vi "CVT1NamedWriteTest.vi"() -> (3 "Unit Test Framework Results":T1)   [LabVIEW 2013, in "UnitTests.lvlib"]
uses:
  UnitTests.lvlib
  <vilib>/utf/common/utf_test_result_troll.ctl
  <vilib>/utf/common/utf_test_result.ctl
  <vilib>/utf/common/utf_test_result_failure.ctl
  <vilib>/utf/common/utf_test_comparison_operators.ctl
  <vilib>/utf/common/utf_vi_tag.ctl
  <vilib>/NI/Current Value Table/Write.vi
  <vilib>/NI/Current Value Table/DataTypes/I32_Write.vi
  <vilib>/NI/Current Value Table/Read.vi
  <vilib>/NI/Current Value Table/DataTypes/I32_Read.vi
  <vilib>/NI/Current Value Table/Type to Enum.vi
  <vilib>/NI/Current Value Table/DataTypes/I32_Type To Enum.vi
  <vilib>/NI/Current Value Table/Compatibility/TagConverter.vi
  <vilib>/NI/Current Value Table/Create Tags.vi
  <vilib>/NI/Current Value Table/FGVs/CVT Globals.vi
  <vilib>/NI/Current Value Table/FGVs/Tag Memory.vi
  <vilib>/NI/Current Value Table/Memory Block.vi
  <vilib>/NI/Current Value Table/DataTypes/I32_Memory Block.vi
  <vilib>/utf/NI_UnitTestFramework.lvlib
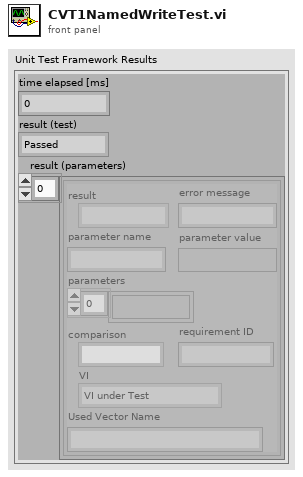
[diagram p1: front panel]
types:
  T1 = typedef "NI_UnitTestFramework.lvlib/utf_test_result_troll.ctl" = cluster{"time elapsed [ms]":u32, "result (test)":T2, "result (parameters)":T3[]}
  T2 = typedef "NI_UnitTestFramework.lvlib/utf_test_result.ctl" = enum16{"Passed", "Failed", "Error", "Skipped", "Not Processed"}
  T3 = typedef "NI_UnitTestFramework.lvlib/utf_test_result_failure.ctl" = cluster{"result":T2, "error message":string, "parameter name":string, "parameter value":variant, "parameters":variant[], "comparison":T4, "requirement ID":string, "VI":T5, "Used Vector Name":string}
  T4 = typedef "NI_UnitTestFramework.lvlib/utf_test_comparison_operators.ctl" = enum16{"=", "!=", ">", ">=", "<", "<=", "range", "symmetric tolerance", "asymmetric tolerance", "string contains", "string not contain", "array size", "string length", "array range", "by element", "array range (limit array)", "user-defined", "array contains", "array not contain", "vector length", "= (elm)", "!= (elm)", "= (case insensitive)", "!= (case insensitive)"}
  T5 = typedef "NI_UnitTestFramework.lvlib/utf_vi_tag.ctl" = enum16{"Setup VI", "VI under Test", "Teardown VI"}
  T6 = typedef "cvt_Tag Configuration.ctl" = cluster{"Name":string, "Data Type":T7, "Array":bool, "Size":u32, "Default":string, "Enum":string[], "Description":string}
  T7 = typedef "cvt_Data Types.ctl" = enum16{"Bool", "U8", "I32", "Double", "String", "Enum"}
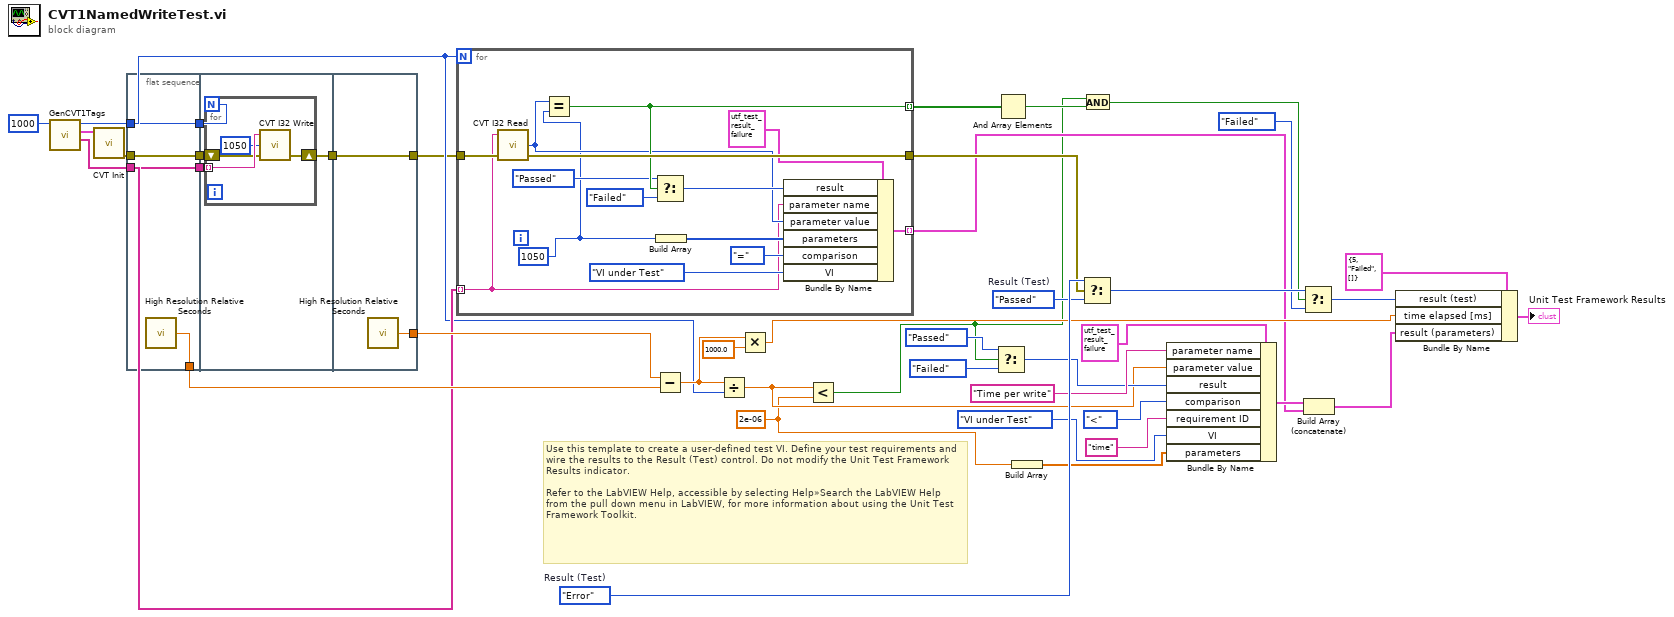
[diagram p0: block diagram]
diagram:
  w5 = 2e-06 ("y")
  w36 = utf_test_result."Error"  # Result (Test)
  w35 = utf_test_result."Passed"  # Result (Test)
  # "Use this template to create a user-defined test VI. Define your test requirements and wire the results to the Result (Test) control. Do not modify the Unit Test Framework Results indicator. \n\nRefer to the LabVIEW Help, accessible by selecting Help»Search the LabVIEW Help from the pull down menu in LabVIEW, for more information about using the Unit Test Framework Toolkit."
  n1 = call "GenCVT1Tags.vi"("Number of Tags in"=1000) -> ("Names"=w21:string[], "Tags"=w29:T6[], "Number of Tags out"=w20:i32)  [unwired: 8 in]
  n2 = call <vilib>:"CVT Init.vi"("Tag List"=w29) -> ("error out"=w28:errorcluster)  [unwired: 10 in]
  n3 = flat-sequence {
    tunnel: [w45] -> w38
    tunnel: w28 -> [w42]
    tunnel: [w44] -> w27
    tunnel: w20 -> [w44]
    tunnel: w21 -> [w43]
    tunnel: [w43] -> w26
    tunnel: [w42] -> w25
    tunnel: w27 -> [w49]
    tunnel: w26 -> [w48]
    tunnel: w25 -> [w47]
    tunnel: [w46] -> w24
    tunnel: [w55] -> w39
    tunnel: w24 -> [w54]
    tunnel: [w54] -> w19
    frame #0 {
      n4 = call <vilib>:"High Resolution Relative Seconds.vi"() -> ("relative seconds"=w45:dbl)
    }
    frame #1 {
      n5 = for {
        N: w49 -> [_]
        tunnel: w48 -> [w53] mode=indexing
        shift-right: [w51] -> w46
        shift-left: w47 -> [w52]
        n6 = call <vilib>:"CVT I32 Write.vi"("error in (no error)"=w52, "Value"=1050, "Tag Name"=w53) -> ("error out"=w51:errorcluster)  [unwired: 2 in]
      }
    }
    frame #2 {
      n7 = call <vilib>:"High Resolution Relative Seconds.vi"() -> ("relative seconds"=w55:dbl)
    }
  }
  n8 = for {
    N: w20 -> [_]
    tunnel: w21 -> [w57] mode=indexing
    tunnel: w19 -> [w69]
    tunnel: [w68] -> w18
    tunnel: [w65] -> w17 mode=indexing
    tunnel: [w61] -> w3 mode=indexing
    w56 = 1050 ("Value")
    n9 = call <vilib>:"CVT I32 Read.vi"("error in (no error)"=w69, "Tag Name"=w57) -> ("error out"=w68:errorcluster, "Value"=w58:i32)  [unwired: 2 in]
    n10 = Equal?(x=w58, y=w56) -> (x = y?=w65:bool)
    n11 = Select(t=utf_test_result."Passed" ("result"), s=w65, f=utf_test_result."Failed" ("result")) -> (s? t:f=w62:T2)
    n12 = Build Array(w56) -> (w59:i32[])
    n13 = Bundle By Name(cluster=T3 {"result"=enum."Passed", "error message"="", "parameter name"="", "parameter value"=variant, "parameters"=[], "comparison"=enum."=", "requirement ID"="", "VI"=enum."Setup VI", "Used Vector Name"=""} ("Unit Test Framework - result (parameters)"), "result"=w62, "parameter name"=w57, "parameter value"=w58, "parameters"=w59, "comparison"=utf_test_comparison_operators."=", "VI"=utf_vi_tag."VI under Test") -> (w61:T3)
  }
  n14 = Subtract(x=w39, y=w38) -> (x-y=w23:dbl)
  n15 = Divide(x=w23, y=w20) -> (x/y=w8:dbl)
  n16 = Multiply(x=w23, y=1000.0) -> (x*y=w30:dbl)
  n17 = Less?(x=w8, y=w5) -> (x < y?=w1:bool)
  n18 = Select(t=utf_test_result."Passed" ("result"), s=w1, f=utf_test_result."Failed" ("result")) -> (s? t:f=w9:T2)
  n19 = And Array Elements(Boolean array=w17) -> (logical AND=w16:bool)
  n20 = Build Array(w5) -> (w4:dbl[])
  n21 = Select(t=w36, s=w18, f=w35) -> (s? t:f=w15:T2)
  n22 = And(x=w1, y=w16) -> (x .and. y?=w2:bool)
  n23 = Bundle By Name(cluster=T3 {"result"=enum."Passed", "error message"="", "parameter name"="", "parameter value"=variant, "parameters"=[], "comparison"=enum."=", "requirement ID"="", "VI"=enum."Setup VI", "Used Vector Name"=""} ("Unit Test Framework - result (parameters)"), "parameter name"="Time per write", "parameter value"=w8, "result"=w9, "comparison"=utf_test_comparison_operators."<", "requirement ID"="time", "VI"=utf_vi_tag."VI under Test", "parameters"=w4) -> (w33:T3)
  n24 = Select(t=w15, s=w2, f=utf_test_result."Failed") -> (s? t:f=w13:T2)
  n25 = Build Array (concatenate)(w33, w3) -> (w32:T3[])
  n26 = Bundle By Name(cluster=T1 {"time elapsed [ms]"=5, "result (test)"=enum."Failed", "result (parameters)"=[]} ("Unit Test Framework - Result"), "result (test)"=w13, "time elapsed [ms]"=w30, "result (parameters)"=w32) -> (→"Unit Test Framework Results":T1)
